vi "Shift.vi"(10 "Confirmação":bool, 11 "DataIn":T4) -> (0 "Turno":string, 1 "Tabuleiro":T1, 3 "DataOut":T2)   [LabVIEW 2017]
doc: "SubVi criada para controlar a troca de turnos entre jogadores durante uma partida."
uses:
  controls/DataIn.ctl
  controls/Tabuleiro.ctl
  controls/GameOption.ctl
  controls/DataOut.ctl
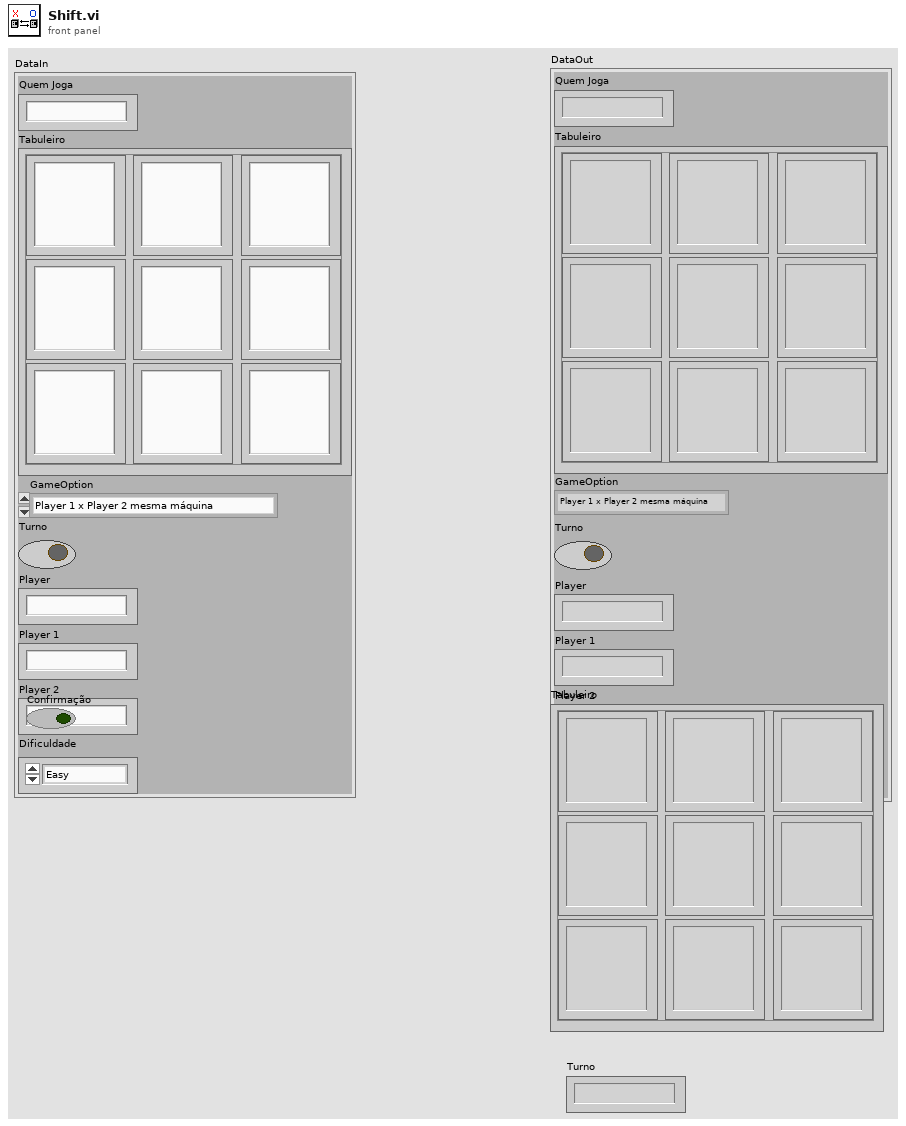
[diagram p1: front panel]
types:
  T1 = typedef "Tabuleiro.ctl" = cluster{"(0,0)":string, "(1,0)":string, "(0,1)":string, "(1,1)":string, "(2,0)":string, "(1,2)":string, "(2,2)":string, "(0,2)":string, "(2,1) ":string}
  T2 = typedef "DataOut.ctl" = cluster{"Quem Joga":string, "Tabuleiro":T1, "GameOption":T3, "Turno":bool, "Player":string, "Player 1":string, "Player 2":string, "Dificuldade":enum16{"Easy", "Medium", "Hard"}}
  T3 = typedef "GameOption.ctl" = enum16{"Player 1 x Player 2 mesma máquina", "Player 1 x Player 2 pela rede", "Player 1 x Computador", "Wait for Event", "Initialize", "Stop"}
  T4 = typedef "DataIn.ctl" = cluster{"Quem Joga":string, "Tabuleiro":T1, "GameOption":T3, "Turno":bool, "Player":string, "Player 1":string, "Player 2":string, "Dificuldade":enum16{"Easy", "Medium", "Hard"}}
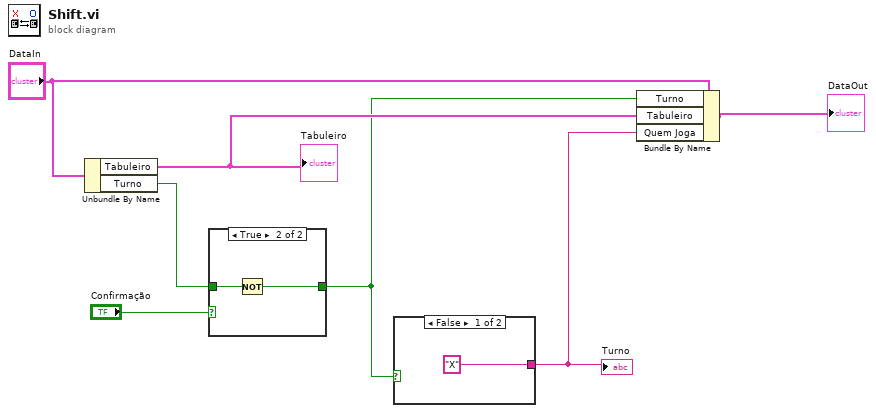
[diagram p0: block diagram]
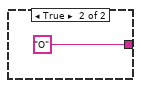
[diagram p2: hidden frame]
diagram:
  n1 = Unbundle By Name("DataIn") -> ("Tabuleiro"=w5:T1, "Turno"=w4:bool)
  "Tabuleiro" <- w5
  n2 = case shown="True" "Confirmação" {
    selector: "Confirmação" -> [w8 _]
    tunnel: [w8 w10] -> w2
    tunnel: w4 -> [_ w9]
    frame False {
    }
    frame True {
      n3 = Not(x=w9) -> (.not. x?=w10:bool)
    }
  }
  n4 = case shown="False" w2 {
    tunnel: ["X" "O"] -> w1
    frame False {
    }
    frame True {
    }
  }
  "Turno" <- w1
  n5 = Bundle By Name(cluster="DataIn", "Turno"=w2, "Tabuleiro"=w5, "Quem Joga"=w1) -> (→"DataOut":T4)
